vi "Run.vi"(11 "Nav6DevRef":T1) -> ()   [LabVIEW 2013, in "Nav6.lvlib"]
uses:
  Nav6.lvlib
  Nav6DevRef.ctl
  <vilib>/Rock Robotics/WPI/SerialPort/WPI_SerialPortRef.ctl
  Nav6Mode.ctl
  StopGlobal.vi
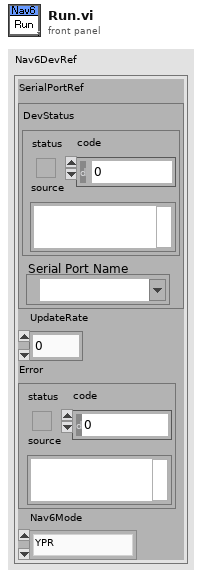
[diagram p1: front panel]
types:
  T1 = typedef "Nav6.lvlib/Nav6DevRef.ctl" = cluster{"SerialPortRef":T2, "UpdateRate":u8, "Error":errorcluster, "Nav6Mode":T3}
  T2 = typedef "WPI_SerialPortRef.ctl" = cluster{"DevStatus":errorcluster, "Serial Port Name":refnum<visa-resource-name>}
  T3 = typedef "Nav6.lvlib/Nav6Mode.ctl" = enum16{"YPR", "Gyro", "Quaternion"}
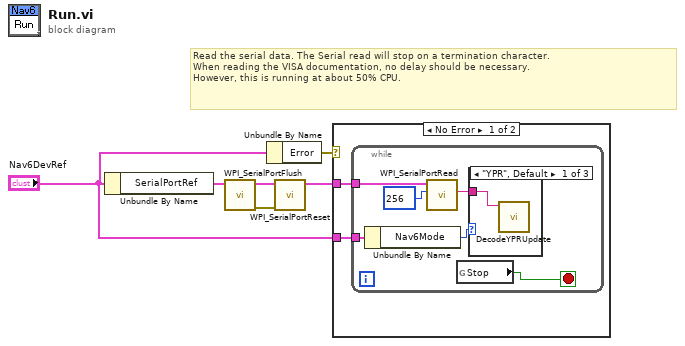
[diagram p0: block diagram]
diagram:
  # "Read the serial data. The Serial read will stop on a termination character.\nWhen reading the VISA documentation, no delay should be necessary. \nHowever, this is running at about 50% CPU."
  n1 = Unbundle By Name("Nav6DevRef") -> ("SerialPortRef"=w3:T2)
  n2 = call <vilib>:"WPI_SerialPortFlush.vi"("SerialPortRef"=w3) -> ("error out"=w6:errorcluster, "SerialPortRef"=w5:T2)  [unwired: 9 in]
  n3 = Unbundle By Name("Nav6DevRef") -> ("Error"=w2:errorcluster)
  n4 = call <vilib>:"WPI_SerialPortReset.vi"("error in (no error)"=w6, "SerialPortRef"=w5) -> ("SerialPortRef"=w4:T2)  [unwired: 8 in, 1 out]
  n5 = case shown="No Error" w2 {
    tunnel: w4 -> [w8 _]
    tunnel: "Nav6DevRef" -> [w7 _]
    frame No Error {
      n6 = while {
        tunnel: w8 -> [w13]
        tunnel: w7 -> [w12]
        stop <- w9 stop-if-true
        n7 = Unbundle By Name(w12) -> ("Nav6Mode"=w11:T3)
        n8 = call <vilib>:"WPI_SerialPortRead.vi"("Num Bytes to Read"=u32 256, "SerialPortRef"=w13) -> ("Buffer"=w14:string)  [unwired: 7 in, 2 out]
        n9 = global read "StopGlobal.vi" "Stop"() -> (w9:bool)
        n10 = case shown="\"YPR\", Default" w11 {
          tunnel: w14 -> [w15 _ _]
          frame "YPR", Default {
            n11 = call "DecodeYPRUpdate.vi"("Buffer"=w15) -> ()  [unwired: 11 in]
          }
          frame "Gyro" {
          }
          frame "Quaternion" {
          }
        }
      }
    }
    frame Error {
    }
  }
